vi "未命名 2.vi"() -> ()   [LabVIEW 2014]
panel:
  out "信号":dbl
  out "Array of Waveform":waveform(dbl)[](array[waveform]) caption="波形数组"
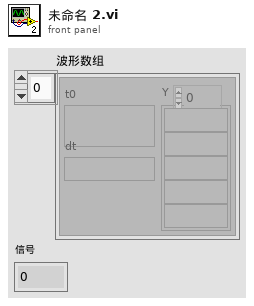
[diagram p1: front panel]
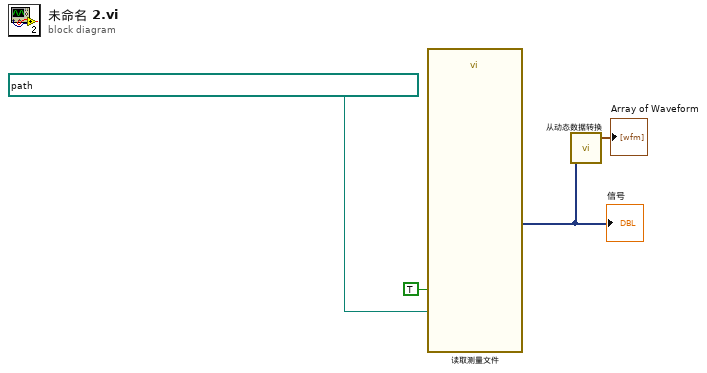
[diagram p0: block diagram]
diagram:
  n1 = call "读取测量文件"("Filename"=path "C:/Users/Administrator/Desktop/自主泊车系统/abc.lvm", "Enable"=TRUE) -> ("Signals"=w2:dynamicdata)  [unwired: 4 in, 5 out]
  "信号" <- w2
  n2 = call "从动态数据转换"("Dynamic Data Type"=w2) -> ("Array of Waveform"=→"Array of Waveform":waveform(dbl)[])  [unwired: 3 in]
